vi "Set DO Status - Multiple.vi"(0 "reference in":refnum<class "DO.lvclass">, 2 "DO Channel Number (Zero Based)":i32[](array[numeric]), 4 "DO Status To Set":bool[](array[boolean]), 5 "error in (no error)":errorcluster) -> (14 "reference out":refnum<class "DO.lvclass">, 16 "DO Channel Number (Zero Based) OUT":i32[](array[numeric]), 19 "error out":errorcluster)   [LabVIEW 2017, in "DO.lvclass"]
uses:
  DO.lvclass
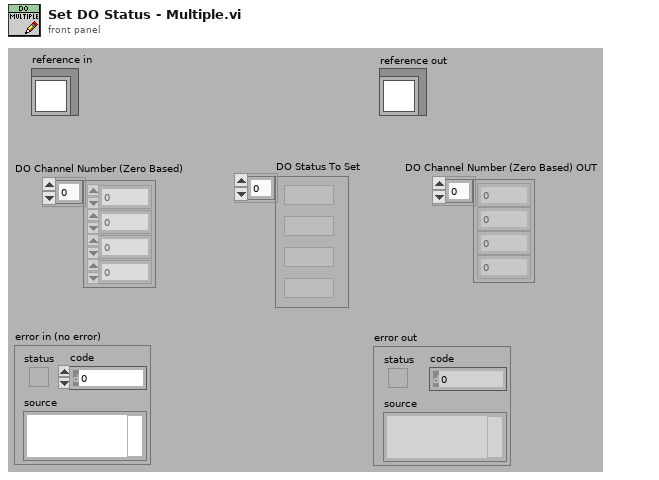
[diagram p1: front panel]
types:
  T1 = typedef "DO.lvclass/ObjectAttributes.ctl" = cluster{"DO Task":refnum<k21>, "DO Module Names (NI-Max Name)":string[], "Number of Channels Per DO Module":i32[], "DO Status":bool[], "Number of DO Modules":u32, "DO Status to Set":bool[], "DO On/Off Status":bool, "DO VI Reference":refnum<vi>, "Number of Total DO Channels":u32}
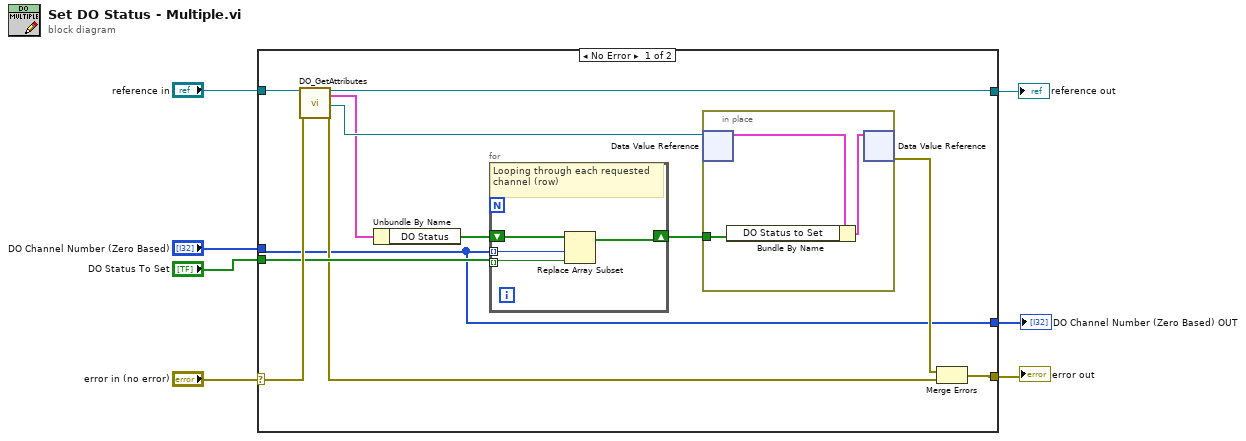
[diagram p0: block diagram]
diagram:
  n1 = case shown="No Error" "error in (no error)" {
    selector: "error in (no error)" -> [w18 w28]
    tunnel: [w15 w28] -> w6
    tunnel: [w16 w27] -> w4
    tunnel: "reference in" -> [w19 w27]
    tunnel: "DO Channel Number (Zero Based)" -> [w8 _]
    tunnel: "DO Status To Set" -> [w11 _]
    tunnel: [w8 _] -> w1
    frame No Error {
      n2 = call "DO_GetAttributes.vi"("reference in"=w19, "error in (no error)"=w18) -> ("reference out"=w16:refnum<class "DO.lvclass">, "Data"=w12:T1, "DataRef"=w14:refnum<data-value>, "error out"=w9:errorcluster)  [unwired: 14 in]
      n3 = Unbundle By Name(w12) -> ("DO Status"=w13:bool[])
      n4 = for {
        tunnel: w8 -> [w23] mode=indexing
        tunnel: w11 -> [w22] mode=indexing
        shift-right: [w20] -> w10
        shift-left: w13 -> [w21]
        # "Looping through each requested channel (row)"
        n5 = Replace Array Subset(array=w21, new element=w22, index=w23) -> (w20:bool[])
      }
      n6 = in-place {
        in-place-border: w10 -> [w24]
        n7 = in-place-dvr #1(w14) -> (w26:T1)  [unwired: 1 out]
        n8 = Bundle By Name(cluster=w26, "DO Status to Set"=w24) -> (w25:T1)
        n9 = in-place-dvr #1(w25) -> (w17:errorcluster)  [unwired: 1 out]
      }
      n10 = Merge Errors(w17, w9) -> (w15:errorcluster)
    }
    frame Error {
    }
  }
  "error out" <- w6
  "reference out" <- w4
  "DO Channel Number (Zero Based) OUT" <- w1
